vi "Launcher.vi"   [LabVIEW 2020]
uses:
  Actor Tests/Actor Tests.lvclass
  C:/Program Files (x86)/National Instruments/LabVIEW 2020/vi.lib/ActorFramework/Actor/Actor.lvclass
  <vilib>/ActorFramework/Actor/Actor.lvclass
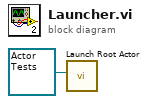
[diagram p0: block diagram]
diagram:
  n1 = call <vilib>:"Launch Root Actor.vi"("Actor"=refnum<class "Actor Tests.lvclass"> refnum ("Actor Tests.lvlib:Actor Tests.lvclass")) -> ()  [unwired: 9 in, 2 out]
